vi "Channels to Block Conversions.vi"(9 "initial engine buffer offset":u64 format="%d bytes", 10 "initial string buffer offset":u64 format="%d bytes", 11 "Transfer Configuration":T1 {"channels"."string offset" format="%d bytes"}) -> (3 "Transfer conversion descriptors":T6[](array[typedef]) {"string offset" format="%d bytes"; "engine offset" format="%d bytes"})   [LabVIEW 2017, in "DSF Core.lvlib" / "DSF Buffer Converter.lvclass"]
uses:
  DSF Buffer Converter.lvclass
  Conversion Block.ctl
  Typedefs/DSF Data Type.ctl
  Typedefs/DSF Engine Transfer Configuration.ctl
  Typedefs/DSF Byte Order.ctl
  Typedefs/DSF Settings Info.ctl
  Typedefs/DSF Engine Channel Configuration.ctl
  Classes/Framework/Framework.lvclass
  DSF Core.lvlib
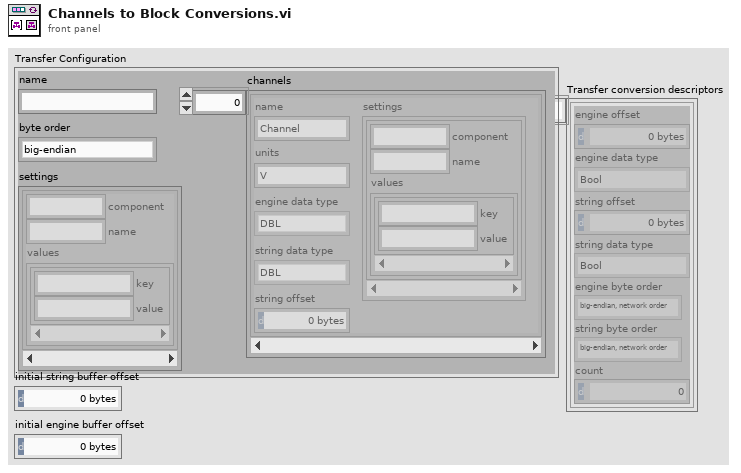
[diagram p1: front panel]
types:
  T1 = typedef "DSF Core.lvlib/DSF Engine Transfer Configuration.ctl" = cluster{"name":string, "byte order":T2, "settings":T3, "channels":T4[]}
  T2 = typedef "DSF Core.lvlib/DSF Byte Order.ctl" = enum8{"big-endian", "little-endian"}
  T3 = typedef "DSF Core.lvlib/DSF Settings Info.ctl" = cluster{"component":string, "name":string, "values":cluster{"key":string, "value":string}[]}[]
  T4 = typedef "DSF Core.lvlib/DSF Engine Channel Configuration.ctl" = cluster{"string offset":u64, "name":string, "units":string, "engine data type":T5, "string data type":T5, "settings":T3}
  T5 = typedef "DSF Core.lvlib/DSF Data Type.ctl" = enum8{"Bool", "SGL", "DBL", "I8", "I16", "I32", "I64", "U8", "U16", "U32", "U64"}
  T6 = typedef "DSF Core.lvlib/DSF Buffer Converter.lvclass/Conversion Block.ctl" = cluster{"engine offset":u64, "engine data type":T5, "string offset":u64, "string data type":T5, "engine byte order":enum16{"big-endian, network order", "native, host order", "little-endian"}, "string byte order":enum16{"big-endian, network order", "native, host order", "little-endian"}, "count":u64}
  T7 = enum16{"big-endian, network order", "native, host order", "little-endian"}
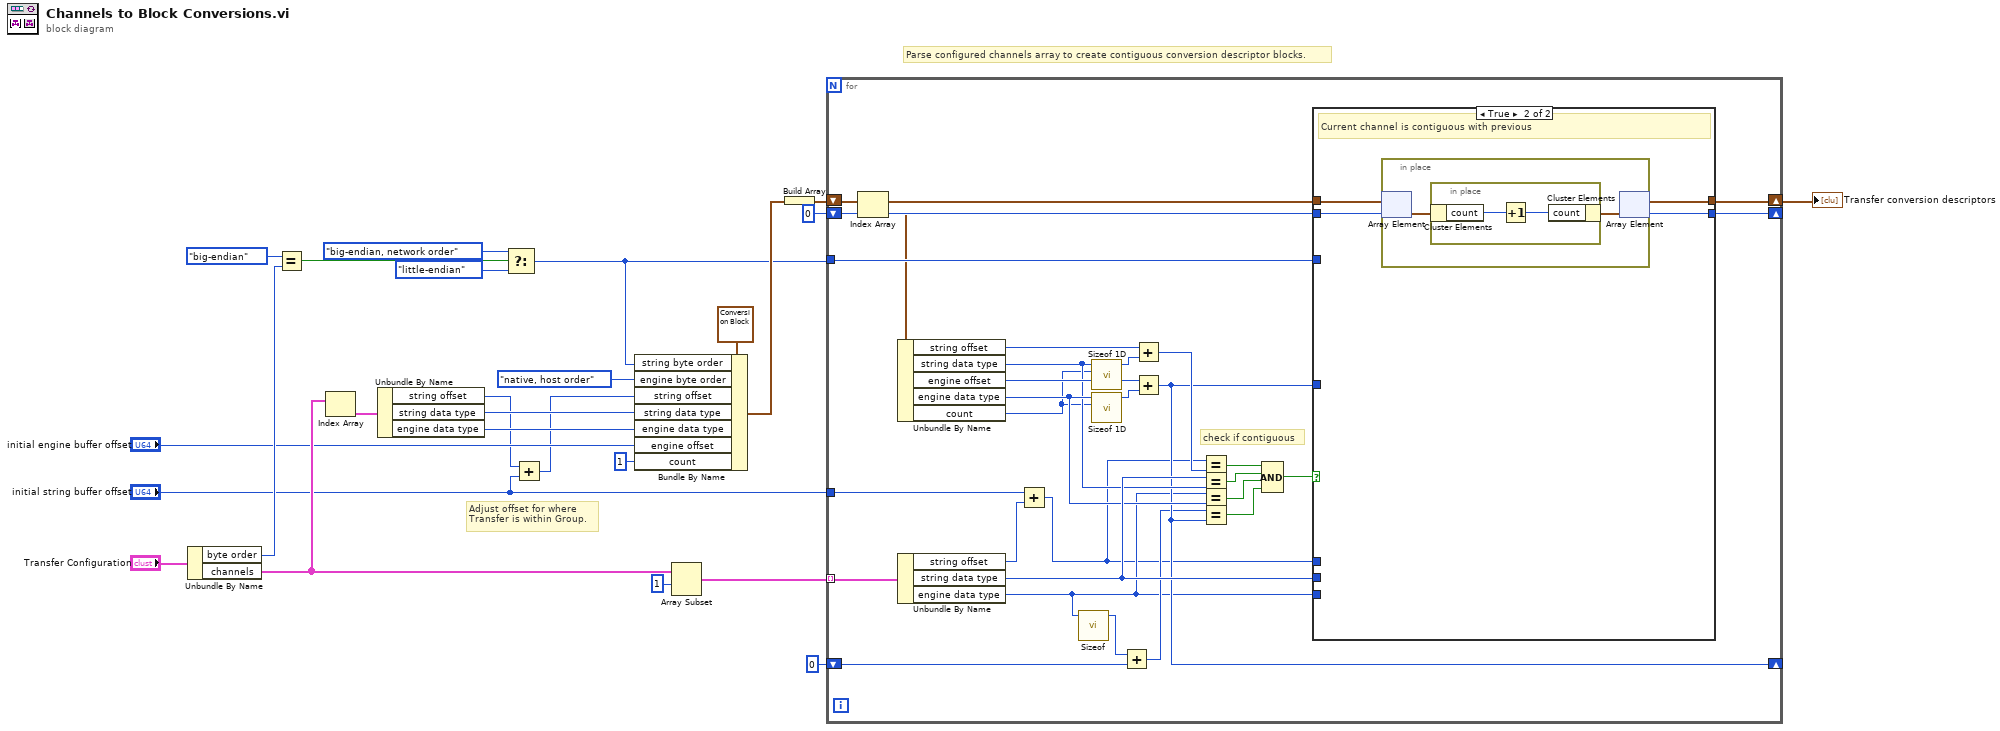
[diagram p0: block diagram]
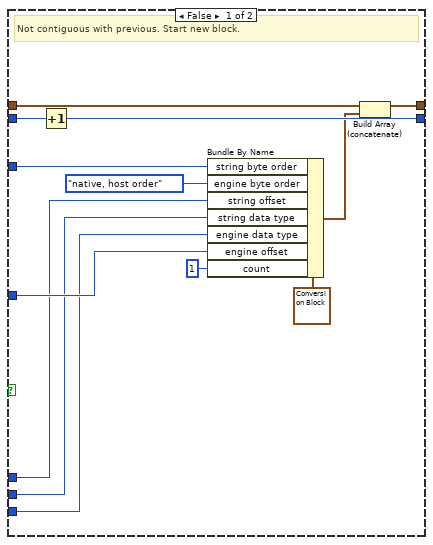
[diagram p2: hidden frame]
diagram:
  # "Adjust offset for where Transfer is within Group."
  # "Parse configured channels array to create contiguous conversion descriptor blocks."
  n1 = Unbundle By Name("Transfer Configuration") -> ("byte order"=w20:T2, "channels"=w13:T4[])
  n2 = Equal?(x=DSF_Byte_Order."big-endian", y=w20) -> (x = y?=w24:bool)
  n3 = Index Array(array=w13) -> (element=w12:T4)  [unwired: 1 in]
  n4 = Unbundle By Name(w12) -> ("string offset"=w1:u64, "string data type"=w14:T5, "engine data type"=w8:T5)
  n5 = Select(t=T7."big-endian, network order" ("engine byte order"), s=w24, f=T7."little-endian" ("engine byte order")) -> (s? t:f=w4:T7)
  n6 = Add(x=w1, y="initial string buffer offset") -> (x+y=w2:u64)
  n7 = Bundle By Name(cluster=T6 {"engine offset"=0, "engine data type"=enum."Bool", "string offset"=0, "string data type"=enum."Bool", "engine byte order"=enum."big-endian, network order", "string byte order"=enum."big-endian, network order", "count"=0} ("conversion descriptor"), "string byte order"=w4, "engine byte order"=T7."native, host order", "string offset"=w2, "string data type"=w14, "engine data type"=w8, "engine offset"="initial engine buffer offset", "count"=u64 1) -> (w5:T6)
  n8 = Array Subset(array=w13, index=1) -> (w15:T4[])  [unwired: 1 in]
  n9 = Build Array(w5) -> (w9:T6[])
  n10 = for {
    tunnel: w15 -> [w54] mode=indexing
    tunnel: w4 -> [w53]
    shift-right: [w34] -> _
    shift-left: u64 0 -> [w31]
    shift-right: [w39] -> w11
    shift-left: w9 -> [w37]
    shift-right: [w38] -> _
    shift-left: 0 -> [w36]
    tunnel: "initial string buffer offset" -> [w28]
    # "check if contiguous"
    n11 = Index Array(array=w37, index=w36) -> (element=w35:T6)
    n12 = Unbundle By Name(w35) -> ("string offset"=w51:u64, "string data type"=w40:T5, "engine offset"=w41:u64, "engine data type"=w42:T5, "count"=w33:u64)
    n13 = Unbundle By Name(w54) -> ("string offset"=w27:u64, "string data type"=w43:T5, "engine data type"=w29:T5)
    n14 = Add(x=w28, y=w27) -> (x+y=w26:u64)
    n15 = call "Sizeof.vi"("data type"=w29) -> ("size in bytes"=w32:u64)  [unwired: 9 in, 1 out]
    n16 = call "Sizeof 1D.vi"("count"=w33, "data type"=w40) -> ("size in bytes"=w50:u64)  [unwired: 9 in]
    n17 = call "Sizeof 1D.vi"("count"=w33, "data type"=w42) -> ("size in bytes"=w52:u64)  [unwired: 9 in]
    n18 = Add(x=w32, y=w31) -> (x+y=w30:u64)
    n19 = Add(x=w51, y=w50) -> (x+y=w49:u64)
    n20 = Add(x=w41, y=w52) -> (x+y=w34:u64)
    n21 = Equal?(x=w26, y=w49) -> (x = y?=w48:bool)
    n22 = Equal?(x=w43, y=w40) -> (x = y?=w45:bool)
    n23 = Equal?(x=w29, y=w42) -> (x = y?=w46:bool)
    n24 = Equal?(x=w30, y=w34) -> (x = y?=w47:bool)
    n25 = Compound Arithmetic op=AND(w48, w45, w46, w47) -> (w44:bool)
    n26 = case shown="True" w44 {
      tunnel: w29 -> [w61 _]
      tunnel: w43 -> [w60 _]
      tunnel: w26 -> [w62 _]
      tunnel: w34 -> [w63 _]
      tunnel: w53 -> [w65 _]
      tunnel: w37 -> [w57 w71]
      tunnel: [w56 w68] -> w39
      tunnel: w36 -> [w59 w70]
      tunnel: [w58 w69] -> w38
      frame False {
        # "Not contiguous with previous. Start new block."
        n27 = Increment(x=w59) -> (x+1=w58:i32)
        n28 = Bundle By Name(cluster=T6 {"engine offset"=0, "engine data type"=enum."Bool", "string offset"=0, "string data type"=enum."Bool", "engine byte order"=enum."big-endian, network order", "string byte order"=enum."big-endian, network order", "count"=0} ("conversion descriptor"), "string byte order"=w65, "engine byte order"=T7."native, host order", "string offset"=w62, "string data type"=w60, "engine data type"=w61, "engine offset"=w63, "count"=u64 1) -> (w55:T6)
        n29 = Build Array (concatenate)(w57, w55) -> (w56:T6[])
      }
      frame True {
        # "Current channel is contiguous with previous"
        n30 = in-place {
          n31 = in-place-array #1(w71, w70) -> (w72:T6)
          n32 = in-place {
            n33 = in-place-cluster #2(w72) -> ("count"=w75:u64)
            n34 = Increment(x=w75) -> (x+1=w74:u64)
            n35 = in-place-cluster #2("count"=w74) -> (w73:T6)
          }
          n36 = in-place-array #1(w73) -> (w68:T6[], w69:i32)
        }
      }
    }
  }
  "Transfer conversion descriptors" <- w11
